vi "get x And y As Point.vi"(11 "Vector 2D in":refnum<class "Vector 2D.lvclass">) -> (3 "Point":T1)   [LabVIEW 2015, in "Vector 2D.lvclass"]
uses:
  Vector 2D.lvclass
  Math/Point (SGL).ctl
  Vector 2D.lvclass/Vector 2D.ctl
  Math/Math.lvlib
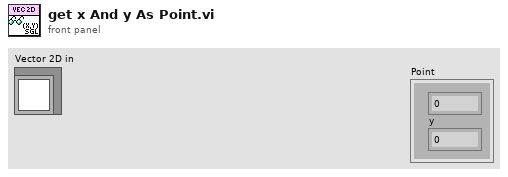
[diagram p1: front panel]
types:
  T1 = typedef "Math.lvlib/Point (SGL).ctl" = cluster{"x":sgl, "y":sgl}
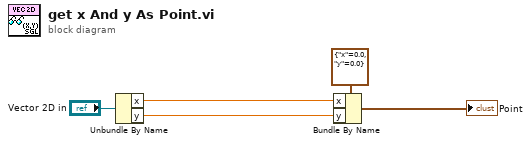
[diagram p0: block diagram]
diagram:
  n1 = Unbundle By Name("Vector 2D in") -> ("x"=w3:sgl, "y"=w2:sgl)
  n2 = Bundle By Name(cluster=T1 {"x"=0.0, "y"=0.0} ("Point"), "x"=w3, "y"=w2) -> (→"Point":T1)
